vi "NotifyIcon - Destroy.vi"(8 "error in":errorcluster, 11 "NotifyIcon reference":refnum<k24>) -> (0 "error out":errorcluster)   [LabVIEW 2018]
doc: "Destroys the NotifyIcon and unregisters any events."
uses:
  System.Windows.Forms
  TypeDefs/NotifyIcon Events.ctl
  TypeDefs/NotifyIcon Event Registration Actions.ctl
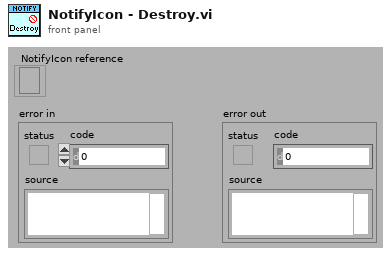
[diagram p1: front panel]
types:
  T1 = typedef "NotifyIcon Event Registration Actions.ctl" = enum16{"Initial Event Registration", "Add to Event Registration", "Destroy Events and Re-register"}
  T2 = typedef "NotifyIcon Events.ctl" = enum16{"BalloonTipClicked", "BalloonTipClosed", "BalloonTipShown", "Click", "Disposed", "DoubleClick", "MouseClick", "MouseDoubleClick", "MouseDown", "MouseMove", "MouseUp", "MenuItemClick", "MenuItemSelect"}
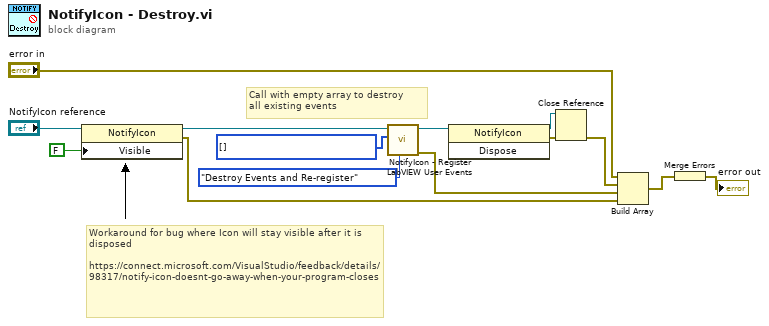
[diagram p0: block diagram]
diagram:
  w7 = T2[] [] items=["BalloonTipClicked", "BalloonTipClosed", "BalloonTipShown", "Click", "Disposed", "DoubleClick", "MouseClick", "MouseDoubleClick", "MouseDown", "MouseMove", "MouseUp", "MenuItemClick", "MenuItemSelect"] ("Events to register")
  # "Call with empty array to destroy\nall existing events"
  # "Workaround for bug where Icon will stay visible after it is disposed\n\nhttps://connect.microsoft.com/VisualStudio/feedback/details/98317/notify-icon-doesnt-go-away-when-your-program-closes"
  n1 = property class="NotifyIcon"(reference="NotifyIcon reference", "Visible"=FALSE) -> (reference out=w9:refnum<k24>, error out=w2:errorcluster)  [unwired: 1 in]
  n2 = call "NotifyIcon - Register LabVIEW User Events.vi"("Action"=NotifyIcon_Event_Registration_Actions."Destroy Events and Re-register", "Events to register"=w7, "NotifyIcon reference in"=w9) -> ("error out"=w3:errorcluster, "NotifyIcon reference out"=w8:refnum<k24>)  [unwired: 6 in, 1 out]
  n3 = invoke class="NotifyIcon" method="Dispose"(reference=w8) -> (reference out=w13:refnum<k24>, error out=w14:errorcluster)  [unwired: 2 in, 1 out]
  n4 = Close Reference(reference=w13, error in (no error)=w14) -> (error out=w4:errorcluster)
  n5 = Build Array("error in", w4, w3, w2) -> (w1:errorcluster[])
  n6 = Merge Errors(w1) -> (→"error out":errorcluster)
